vi "Decode Cordinate with Text.vi"(8 "Error In":errorcluster, 10 "Encoded Cordinate":string) -> (0 "Error Out":errorcluster, 2 "Decoded Cordinate":u32)   [LabVIEW 2022 SP3]
uses:
  <vilib>/Utility/error.llb/Trim Whitespace One-Sided.vi
  <vilib>/regexp/Match Regular Expression.xnode
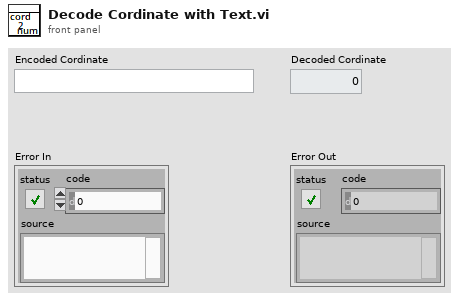
[diagram p1: front panel]
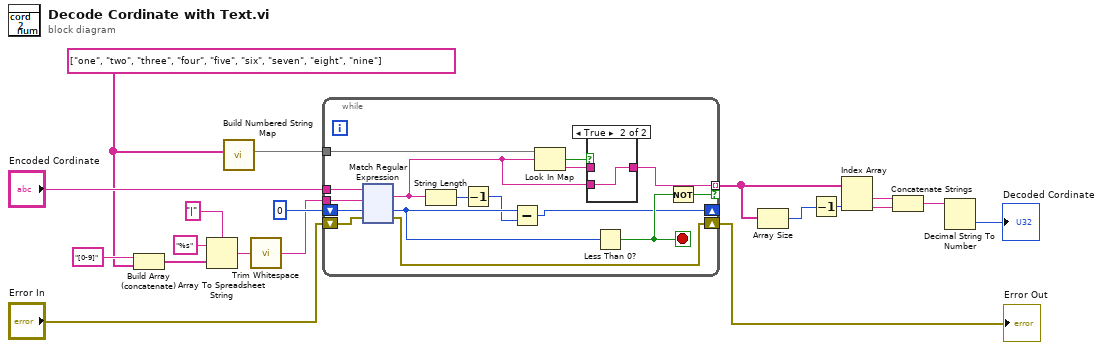
[diagram p0: block diagram]
diagram:
  w4 = string[] ["one", "two", "three", "four", "five", "six", "seven", "eight", "nine"]
  n1 = Build Array (concatenate)("[0-9]", w4) -> (w6:string[])
  n2 = Array To Spreadsheet String(delimiter (Tab)="|", array=w6, 3:"%s" ("format string")) -> (spreadsheet string=w11:string)
  n3 = call "Build Numbered String Map.vi"("Strings"=w4) -> ("Map"=w5:map{string, string})  [unwired: 10 in]
  n4 = call <vilib>:"Trim Whitespace.vi"("string"=w11) -> ("trimmed string"=w3:string)  [unwired: 1 in]
  n5 = while {
    tunnel: "Encoded Cordinate" -> [w32]
    tunnel: [w24] -> w17 mode=indexing if=w34
    shift-right: [w22] -> _
    shift-left: 0 ("offset past match") -> [w31]
    tunnel: w3 -> [w33]
    tunnel: w5 -> [w27]
    shift-right: [w20] -> w1
    shift-left: "Error In" -> [w21]
    stop <- w35 stop-if-true
    n6 = xnode "Match Regular Expression"("input string"=w32, "regular expression"=w33, "offset (0)"=w31, "error in"=w21) -> ("whole match"=w23:string, "offset past match"=w30:i32, "error out"=w20:errorcluster)  [unwired: 2 in, 2 out]
    n7 = String Length(string=w23) -> (length=w29:i32)
    n8 = Decrement(x=w29) -> (x-1=w28:i32)
    n9 = Subtract(x=w30, y=w28) -> (x-y=w22:i32)
    n10 = Look In Map(map=w27, key=w23) -> (key not found?=w26:bool, value=w25:string)  [unwired: 1 in]
    n11 = case shown="True" w26 {
      tunnel: w25 -> [w36 _]
      tunnel: [w36 w37] -> w24
      tunnel: w23 -> [_ w37]
      frame False {
      }
      frame True {
      }
    }
    n12 = Less Than 0?(x=w30) -> (x < 0?=w35:bool)
    n13 = Not(x=w35) -> (.not. x?=w34:bool)
  }
  "Error Out" <- w1
  n14 = Array Size(array=w17) -> (size(s)=w16:i32)
  n15 = Decrement(x=w16) -> (x-1=w15:i32)
  n16 = Index Array(array=w17, index #2=w15) -> (element #1=w10:string, element #2=w9:string)  [unwired: 1 in]
  n17 = Concatenate Strings(w10, w9) -> (w8:string)
  n18 = Decimal String To Number(string=w8) -> (number=→"Decoded Cordinate":i32)  [unwired: 2 in, 1 out]
